vi "TDC_Histogram.vi"(3 "Hist array in":u16[][](array[numeric]), 5 "Data In":cluster{"Channel":u8, "TDC Data":u16}[](array[cluster])) -> (1 "Hist array out":u16[][](array[numeric]))   [LabVIEW 2014]
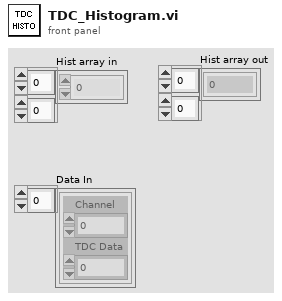
[diagram p1: front panel]
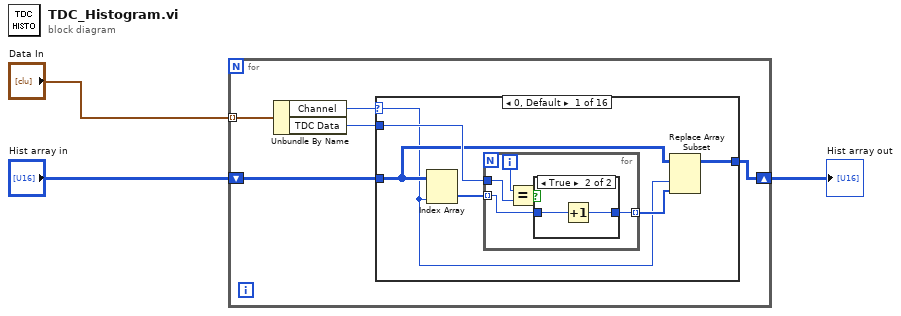
[diagram p0: block diagram]
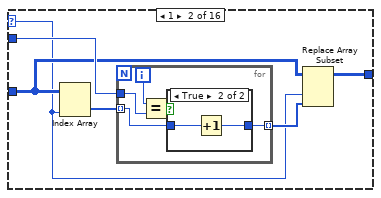
[diagram p3: hidden frame]
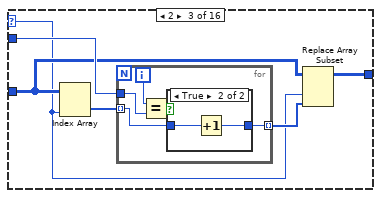
[diagram p5: hidden frame]
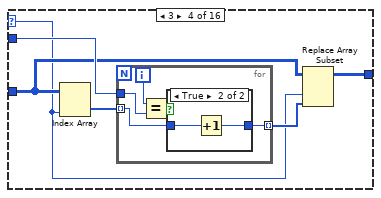
[diagram p7: hidden frame]
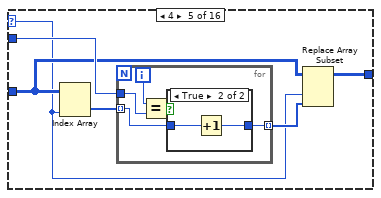
[diagram p9: hidden frame]
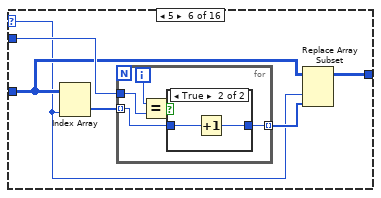
[diagram p11: hidden frame]
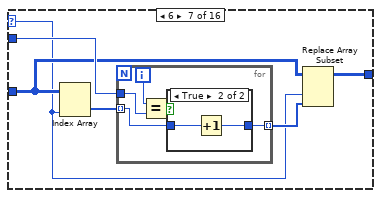
[diagram p13: hidden frame]
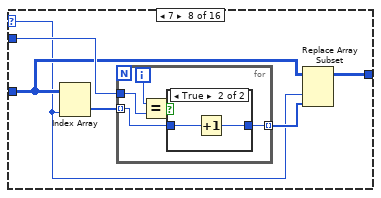
[diagram p15: hidden frame]
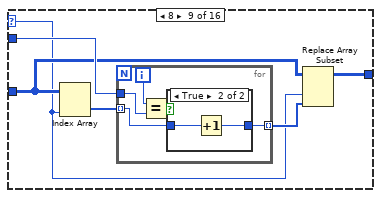
[diagram p17: hidden frame]
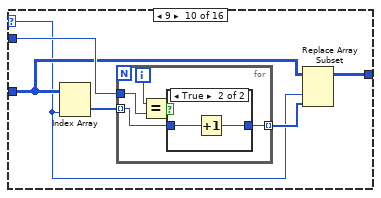
[diagram p19: hidden frame]
diagram:
  n1 = for {
    tunnel: "Data In" -> [w8] mode=indexing
    shift-right: [w4] -> w1
    shift-left: "Hist array in" -> [w5]
    n2 = Unbundle By Name(w8) -> ("Channel"=w7:u8, "TDC Data"=w6:u16)
    n3 = case shown="0, Default" w7 {
      selector: w7 -> [w10 w24 w38 w52 w66 w80 w94 w108 w122 w136 w150 w164 w178 w192 w206 w220]
      tunnel: w6 -> [w13 w27 w41 w55 w69 w83 w97 w111 w125 w139 w153 w167 w181 w195 w209 w223]
      tunnel: w5 -> [w12 w26 w40 w54 w68 w82 w96 w110 w124 w138 w152 w166 w180 w194 w208 w222]
      tunnel: [w9 w23 w37 w51 w65 w79 w93 w107 w121 w135 w149 w163 w177 w191 w205 w219] -> w4
      frame 0, Default {
        n4 = Index Array(array=w12, index (col)=w10) -> (element=w14:u16[])  [unwired: 1 in]
        n5 = for {
          tunnel: w14 -> [w16] mode=indexing
          tunnel: w13 -> [w17]
          tunnel: [w15] -> w11 mode=indexing
          i -> [w18]
          n6 = Equal?(x=w18, y=w17) -> (x = y?=w19:bool)
          n7 = case shown="True" w19 {
            tunnel: w16 -> [w20 w22]
            tunnel: [w20 w21] -> w15
            frame False {
            }
            frame True {
              n8 = Increment(x=w22) -> (x+1=w21:u16)
            }
          }
        }
        n9 = Replace Array Subset(array=w12, new element=w11, index (col)=w10) -> (w9:u16[][])  [unwired: 1 in]
      }
      frame 1 {
        n10 = Index Array(array=w26, index (col)=w24) -> (element=w28:u16[])  [unwired: 1 in]
        n11 = for {
          tunnel: w28 -> [w30] mode=indexing
          tunnel: w27 -> [w31]
          tunnel: [w29] -> w25 mode=indexing
          i -> [w32]
          n12 = Equal?(x=w32, y=w31) -> (x = y?=w33:bool)
          n13 = case shown="True" w33 {
            tunnel: w30 -> [w34 w36]
            tunnel: [w34 w35] -> w29
            frame False {
            }
            frame True {
              n14 = Increment(x=w36) -> (x+1=w35:u16)
            }
          }
        }
        n15 = Replace Array Subset(array=w26, new element=w25, index (col)=w24) -> (w23:u16[][])  [unwired: 1 in]
      }
      frame 2 {
        n16 = Index Array(array=w40, index (col)=w38) -> (element=w42:u16[])  [unwired: 1 in]
        n17 = for {
          tunnel: w42 -> [w44] mode=indexing
          tunnel: w41 -> [w45]
          tunnel: [w43] -> w39 mode=indexing
          i -> [w46]
          n18 = Equal?(x=w46, y=w45) -> (x = y?=w47:bool)
          n19 = case shown="True" w47 {
            tunnel: w44 -> [w48 w50]
            tunnel: [w48 w49] -> w43
            frame False {
            }
            frame True {
              n20 = Increment(x=w50) -> (x+1=w49:u16)
            }
          }
        }
        n21 = Replace Array Subset(array=w40, new element=w39, index (col)=w38) -> (w37:u16[][])  [unwired: 1 in]
      }
      frame 3 {
        n22 = Index Array(array=w54, index (col)=w52) -> (element=w56:u16[])  [unwired: 1 in]
        n23 = for {
          tunnel: w56 -> [w58] mode=indexing
          tunnel: w55 -> [w59]
          tunnel: [w57] -> w53 mode=indexing
          i -> [w60]
          n24 = Equal?(x=w60, y=w59) -> (x = y?=w61:bool)
          n25 = case shown="True" w61 {
            tunnel: w58 -> [w62 w64]
            tunnel: [w62 w63] -> w57
            frame False {
            }
            frame True {
              n26 = Increment(x=w64) -> (x+1=w63:u16)
            }
          }
        }
        n27 = Replace Array Subset(array=w54, new element=w53, index (col)=w52) -> (w51:u16[][])  [unwired: 1 in]
      }
      frame 4 {
        n28 = Index Array(array=w68, index (col)=w66) -> (element=w70:u16[])  [unwired: 1 in]
        n29 = for {
          tunnel: w70 -> [w72] mode=indexing
          tunnel: w69 -> [w73]
          tunnel: [w71] -> w67 mode=indexing
          i -> [w74]
          n30 = Equal?(x=w74, y=w73) -> (x = y?=w75:bool)
          n31 = case shown="True" w75 {
            tunnel: w72 -> [w76 w78]
            tunnel: [w76 w77] -> w71
            frame False {
            }
            frame True {
              n32 = Increment(x=w78) -> (x+1=w77:u16)
            }
          }
        }
        n33 = Replace Array Subset(array=w68, new element=w67, index (col)=w66) -> (w65:u16[][])  [unwired: 1 in]
      }
      frame 5 {
        n34 = Index Array(array=w82, index (col)=w80) -> (element=w84:u16[])  [unwired: 1 in]
        n35 = for {
          tunnel: w84 -> [w86] mode=indexing
          tunnel: w83 -> [w87]
          tunnel: [w85] -> w81 mode=indexing
          i -> [w88]
          n36 = Equal?(x=w88, y=w87) -> (x = y?=w89:bool)
          n37 = case shown="True" w89 {
            tunnel: w86 -> [w90 w92]
            tunnel: [w90 w91] -> w85
            frame False {
            }
            frame True {
              n38 = Increment(x=w92) -> (x+1=w91:u16)
            }
          }
        }
        n39 = Replace Array Subset(array=w82, new element=w81, index (col)=w80) -> (w79:u16[][])  [unwired: 1 in]
      }
      frame 6 {
        n40 = Index Array(array=w96, index (col)=w94) -> (element=w98:u16[])  [unwired: 1 in]
        n41 = for {
          tunnel: w98 -> [w100] mode=indexing
          tunnel: w97 -> [w101]
          tunnel: [w99] -> w95 mode=indexing
          i -> [w102]
          n42 = Equal?(x=w102, y=w101) -> (x = y?=w103:bool)
          n43 = case shown="True" w103 {
            tunnel: w100 -> [w104 w106]
            tunnel: [w104 w105] -> w99
            frame False {
            }
            frame True {
              n44 = Increment(x=w106) -> (x+1=w105:u16)
            }
          }
        }
        n45 = Replace Array Subset(array=w96, new element=w95, index (col)=w94) -> (w93:u16[][])  [unwired: 1 in]
      }
      frame 7 {
        n46 = Index Array(array=w110, index (col)=w108) -> (element=w112:u16[])  [unwired: 1 in]
        n47 = for {
          tunnel: w112 -> [w114] mode=indexing
          tunnel: w111 -> [w115]
          tunnel: [w113] -> w109 mode=indexing
          i -> [w116]
          n48 = Equal?(x=w116, y=w115) -> (x = y?=w117:bool)
          n49 = case shown="True" w117 {
            tunnel: w114 -> [w118 w120]
            tunnel: [w118 w119] -> w113
            frame False {
            }
            frame True {
              n50 = Increment(x=w120) -> (x+1=w119:u16)
            }
          }
        }
        n51 = Replace Array Subset(array=w110, new element=w109, index (col)=w108) -> (w107:u16[][])  [unwired: 1 in]
      }
      frame 8 {
        n52 = Index Array(array=w124, index (col)=w122) -> (element=w126:u16[])  [unwired: 1 in]
        n53 = for {
          tunnel: w126 -> [w128] mode=indexing
          tunnel: w125 -> [w129]
          tunnel: [w127] -> w123 mode=indexing
          i -> [w130]
          n54 = Equal?(x=w130, y=w129) -> (x = y?=w131:bool)
          n55 = case shown="True" w131 {
            tunnel: w128 -> [w132 w134]
            tunnel: [w132 w133] -> w127
            frame False {
            }
            frame True {
              n56 = Increment(x=w134) -> (x+1=w133:u16)
            }
          }
        }
        n57 = Replace Array Subset(array=w124, new element=w123, index (col)=w122) -> (w121:u16[][])  [unwired: 1 in]
      }
      frame 9 {
        n58 = Index Array(array=w138, index (col)=w136) -> (element=w140:u16[])  [unwired: 1 in]
        n59 = for {
          tunnel: w140 -> [w142] mode=indexing
          tunnel: w139 -> [w143]
          tunnel: [w141] -> w137 mode=indexing
          i -> [w144]
          n60 = Equal?(x=w144, y=w143) -> (x = y?=w145:bool)
          n61 = case shown="True" w145 {
            tunnel: w142 -> [w146 w148]
            tunnel: [w146 w147] -> w141
            frame False {
            }
            frame True {
              n62 = Increment(x=w148) -> (x+1=w147:u16)
            }
          }
        }
        n63 = Replace Array Subset(array=w138, new element=w137, index (col)=w136) -> (w135:u16[][])  [unwired: 1 in]
      }
      frame 10 {
        n64 = Index Array(array=w152, index (col)=w150) -> (element=w154:u16[])  [unwired: 1 in]
        n65 = for {
          tunnel: w154 -> [w156] mode=indexing
          tunnel: w153 -> [w157]
          tunnel: [w155] -> w151 mode=indexing
          i -> [w158]
          n66 = Equal?(x=w158, y=w157) -> (x = y?=w159:bool)
          n67 = case shown="True" w159 {
            tunnel: w156 -> [w160 w162]
            tunnel: [w160 w161] -> w155
            frame False {
            }
            frame True {
              n68 = Increment(x=w162) -> (x+1=w161:u16)
            }
          }
        }
        n69 = Replace Array Subset(array=w152, new element=w151, index (col)=w150) -> (w149:u16[][])  [unwired: 1 in]
      }
      frame 11 {
        n70 = Index Array(array=w166, index (col)=w164) -> (element=w168:u16[])  [unwired: 1 in]
        n71 = for {
          tunnel: w168 -> [w170] mode=indexing
          tunnel: w167 -> [w171]
          tunnel: [w169] -> w165 mode=indexing
          i -> [w172]
          n72 = Equal?(x=w172, y=w171) -> (x = y?=w173:bool)
          n73 = case shown="True" w173 {
            tunnel: w170 -> [w174 w176]
            tunnel: [w174 w175] -> w169
            frame False {
            }
            frame True {
              n74 = Increment(x=w176) -> (x+1=w175:u16)
            }
          }
        }
        n75 = Replace Array Subset(array=w166, new element=w165, index (col)=w164) -> (w163:u16[][])  [unwired: 1 in]
      }
      frame 12 {
        n76 = Index Array(array=w180, index (col)=w178) -> (element=w182:u16[])  [unwired: 1 in]
        n77 = for {
          tunnel: w182 -> [w184] mode=indexing
          tunnel: w181 -> [w185]
          tunnel: [w183] -> w179 mode=indexing
          i -> [w186]
          n78 = Equal?(x=w186, y=w185) -> (x = y?=w187:bool)
          n79 = case shown="True" w187 {
            tunnel: w184 -> [w188 w190]
            tunnel: [w188 w189] -> w183
            frame False {
            }
            frame True {
              n80 = Increment(x=w190) -> (x+1=w189:u16)
            }
          }
        }
        n81 = Replace Array Subset(array=w180, new element=w179, index (col)=w178) -> (w177:u16[][])  [unwired: 1 in]
      }
      frame 13 {
        n82 = Index Array(array=w194, index (col)=w192) -> (element=w196:u16[])  [unwired: 1 in]
        n83 = for {
          tunnel: w196 -> [w198] mode=indexing
          tunnel: w195 -> [w199]
          tunnel: [w197] -> w193 mode=indexing
          i -> [w200]
          n84 = Equal?(x=w200, y=w199) -> (x = y?=w201:bool)
          n85 = case shown="True" w201 {
            tunnel: w198 -> [w202 w204]
            tunnel: [w202 w203] -> w197
            frame False {
            }
            frame True {
              n86 = Increment(x=w204) -> (x+1=w203:u16)
            }
          }
        }
        n87 = Replace Array Subset(array=w194, new element=w193, index (col)=w192) -> (w191:u16[][])  [unwired: 1 in]
      }
      frame 14 {
        n88 = Index Array(array=w208, index (col)=w206) -> (element=w210:u16[])  [unwired: 1 in]
        n89 = for {
          tunnel: w210 -> [w212] mode=indexing
          tunnel: w209 -> [w213]
          tunnel: [w211] -> w207 mode=indexing
          i -> [w214]
          n90 = Equal?(x=w214, y=w213) -> (x = y?=w215:bool)
          n91 = case shown="True" w215 {
            tunnel: w212 -> [w216 w218]
            tunnel: [w216 w217] -> w211
            frame False {
            }
            frame True {
              n92 = Increment(x=w218) -> (x+1=w217:u16)
            }
          }
        }
        n93 = Replace Array Subset(array=w208, new element=w207, index (col)=w206) -> (w205:u16[][])  [unwired: 1 in]
      }
      frame 15 {
        n94 = Index Array(array=w222, index (col)=w220) -> (element=w224:u16[])  [unwired: 1 in]
        n95 = for {
          tunnel: w224 -> [w226] mode=indexing
          tunnel: w223 -> [w227]
          tunnel: [w225] -> w221 mode=indexing
          i -> [w228]
          n96 = Equal?(x=w228, y=w227) -> (x = y?=w229:bool)
          n97 = case shown="True" w229 {
            tunnel: w226 -> [w230 w232]
            tunnel: [w230 w231] -> w225
            frame False {
            }
            frame True {
              n98 = Increment(x=w232) -> (x+1=w231:u16)
            }
          }
        }
        n99 = Replace Array Subset(array=w222, new element=w221, index (col)=w220) -> (w219:u16[][])  [unwired: 1 in]
      }
    }
  }
  "Hist array out" <- w1
